vi "ClientRedo.vi"() -> ()   [LabVIEW 2021]
uses:
  20d74f8f-2e8a-4c06-b98a-87e5722cdd8e.vi
  62bce69e-c64b-4137-aa5a-28c05fbbfa3f.vi
  291e4df5-79fb-4e3f-9a4e-f279d7d5f535.vi
  9bb5296f-f4a3-453d-b6f9-cf16bd393dd9.vi
  233518c0-d511-4a3a-97e5-802c987fc087.vi
  913f2bc2-969c-46f7-9a09-9ea84eabe3ee.vi
  <vilib>/Utility/file.llb/Write Delimited Spreadsheet (string).vi
panel:
  in  "file path (dialog if empty)":path=path "D:/APU Stuff/Bachelor of Computer Science (Intelligent Systems) [APD2F2202CS(IS)]/Semester 1/System Programming and Computer Control [CT047-3-2-SPCC]/Assignment/SystemRedo/Zone Status Changes.csv"
  in  "stop":bool
  in  "C6":bool
  in  "C5":bool
  in  "C4":bool
  in  "C3":bool
  in  "C2":bool
  in  "C1":bool
  in  "B6":bool
  in  "B5":bool
  in  "B4":bool
  in  "B3":bool
  in  "B2":bool
  in  "B1":bool
  in  "A6":bool
  in  "A5":bool
  in  "A4":bool
  in  "A3":bool
  in  "A2":bool
  in  "A1":bool
  # "1"
  # "2"
  # "3"
  # "4"
  # "5"
  # "6"
  # "Alarm Switches"
  # "Zone"
  # "Bypass Switches"
  # "Tamper Switches"
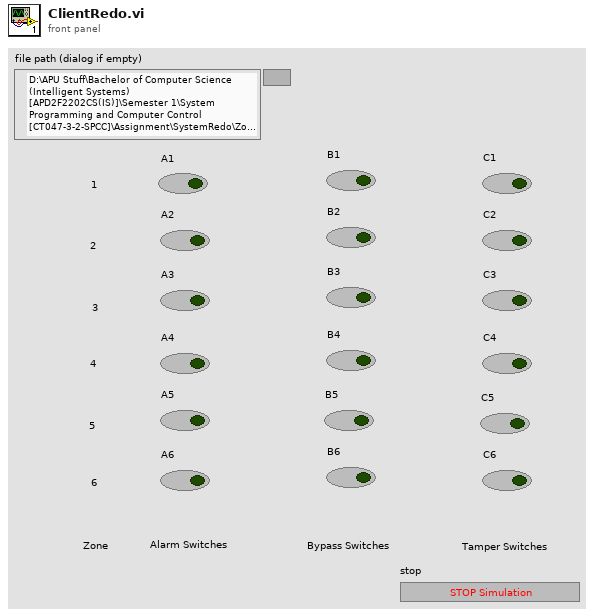
[diagram p1: front panel]
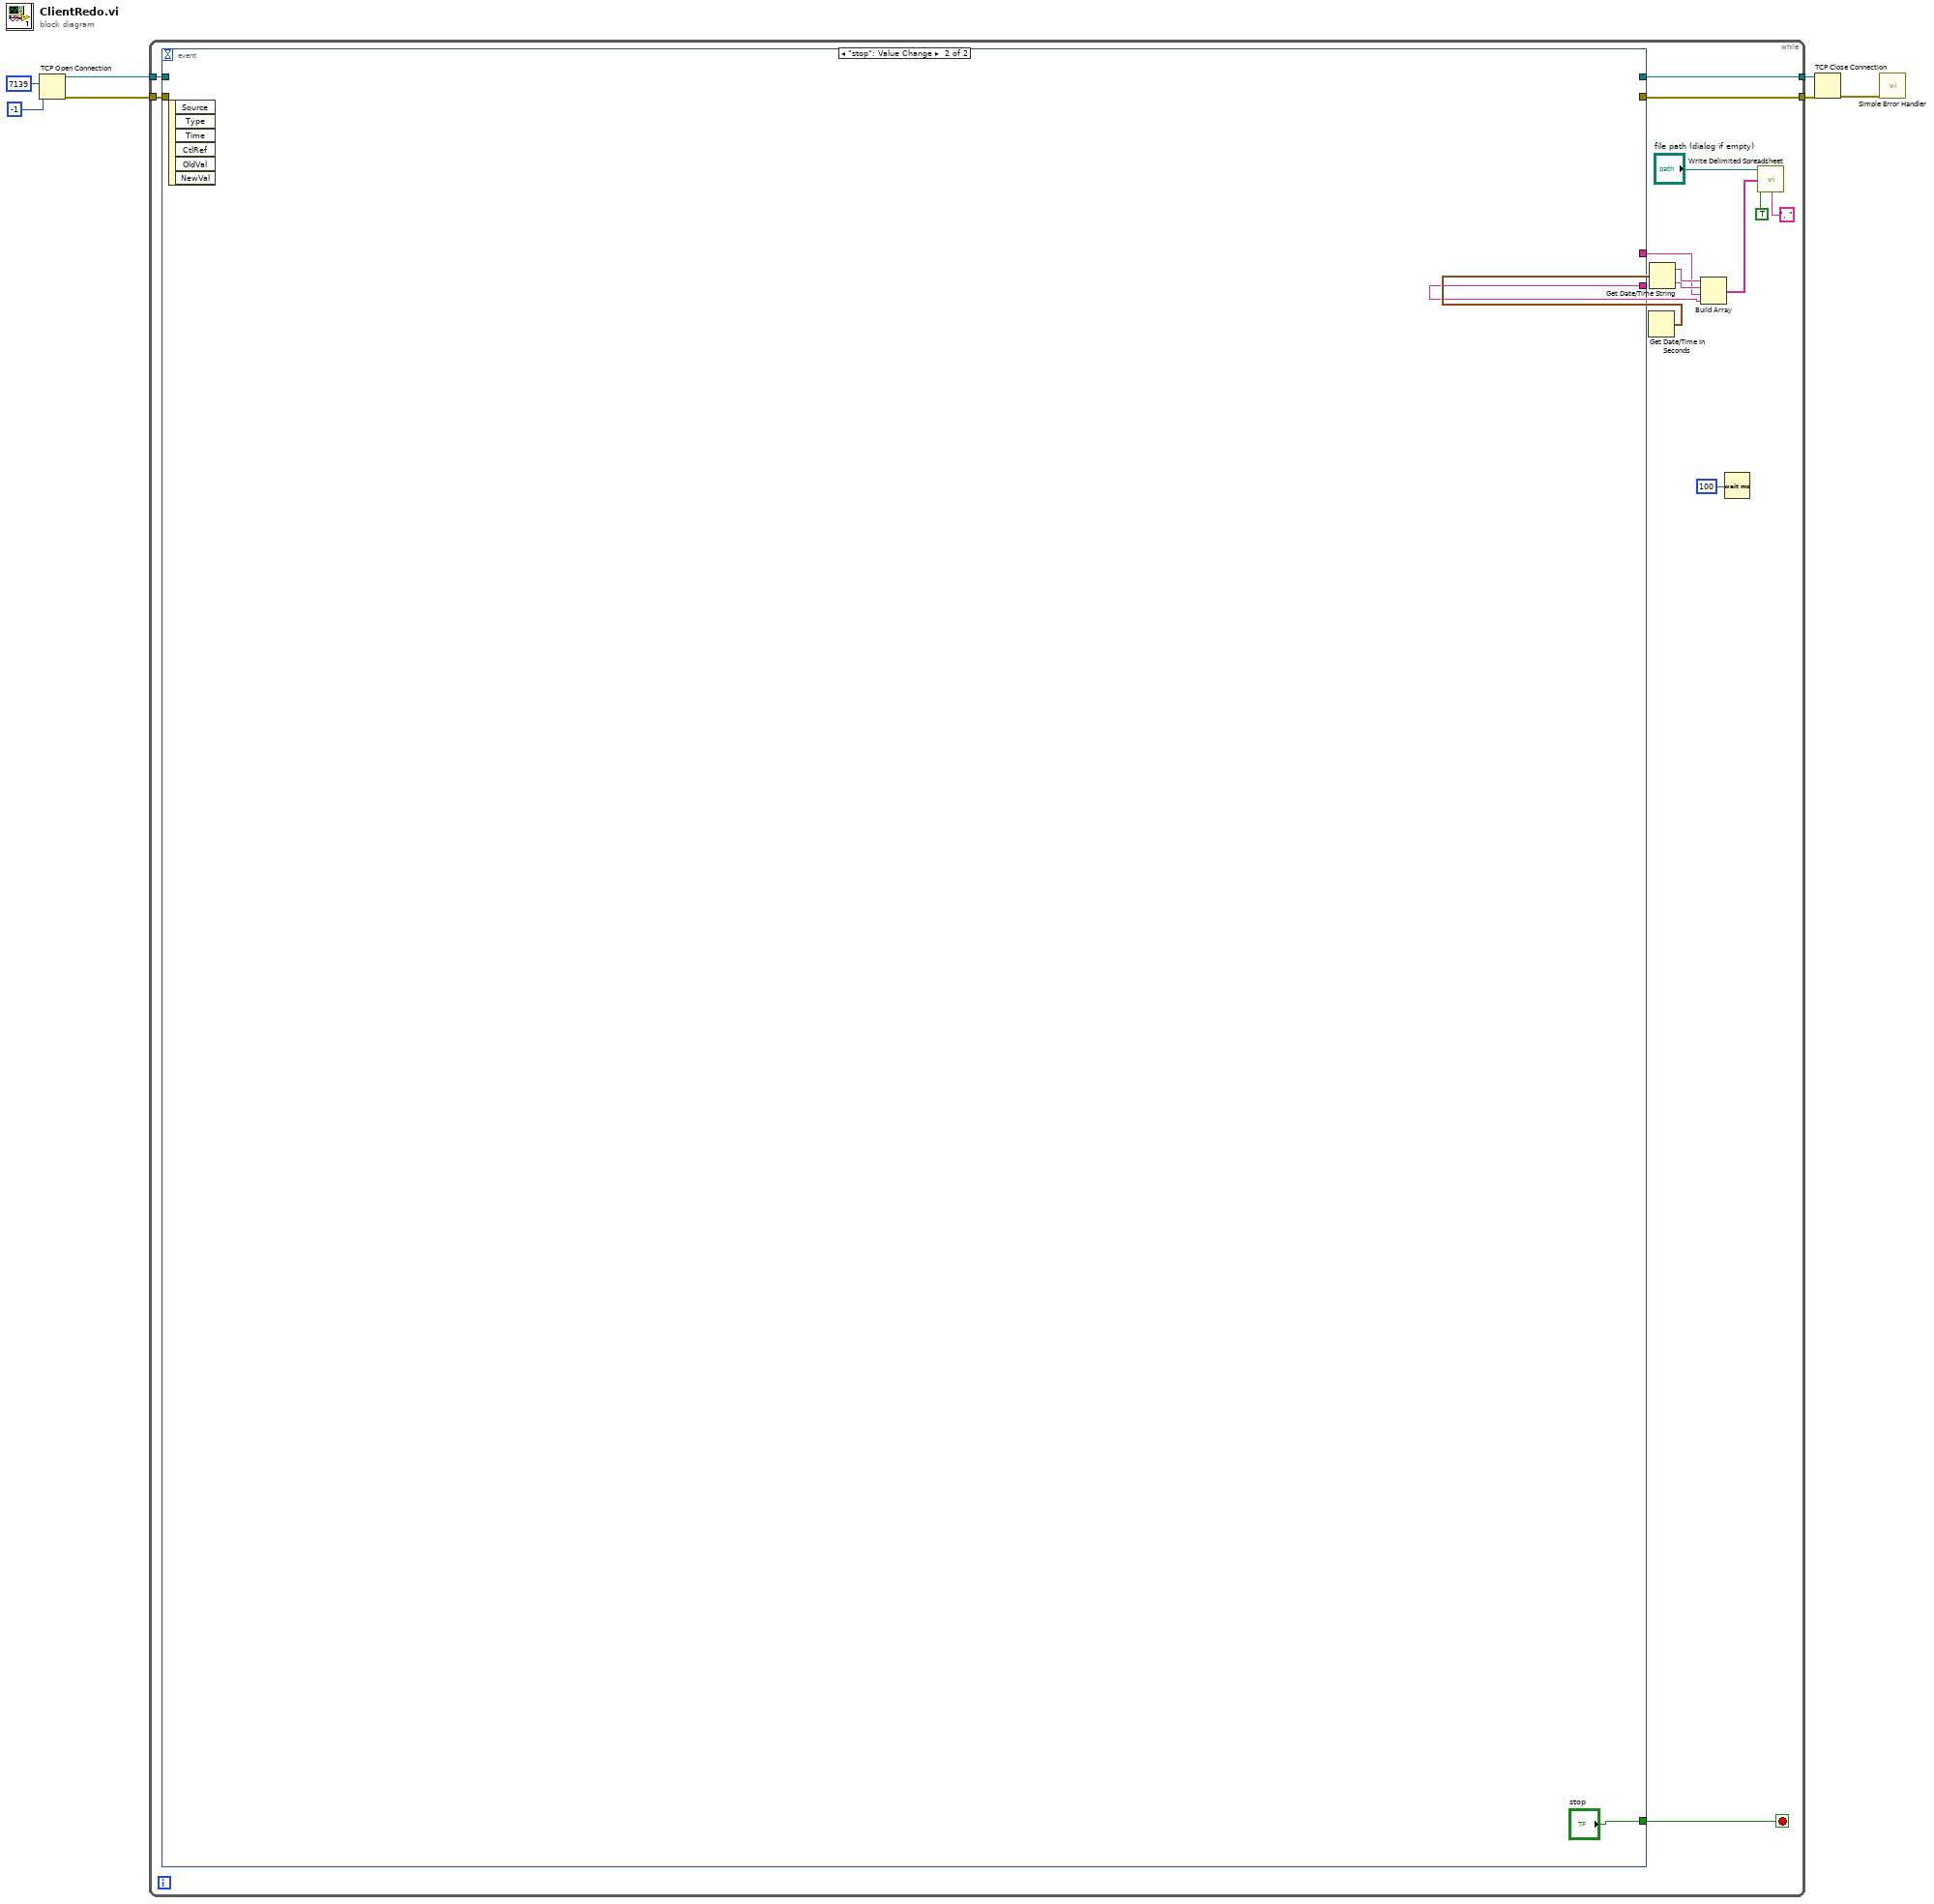
[diagram p0: block diagram]
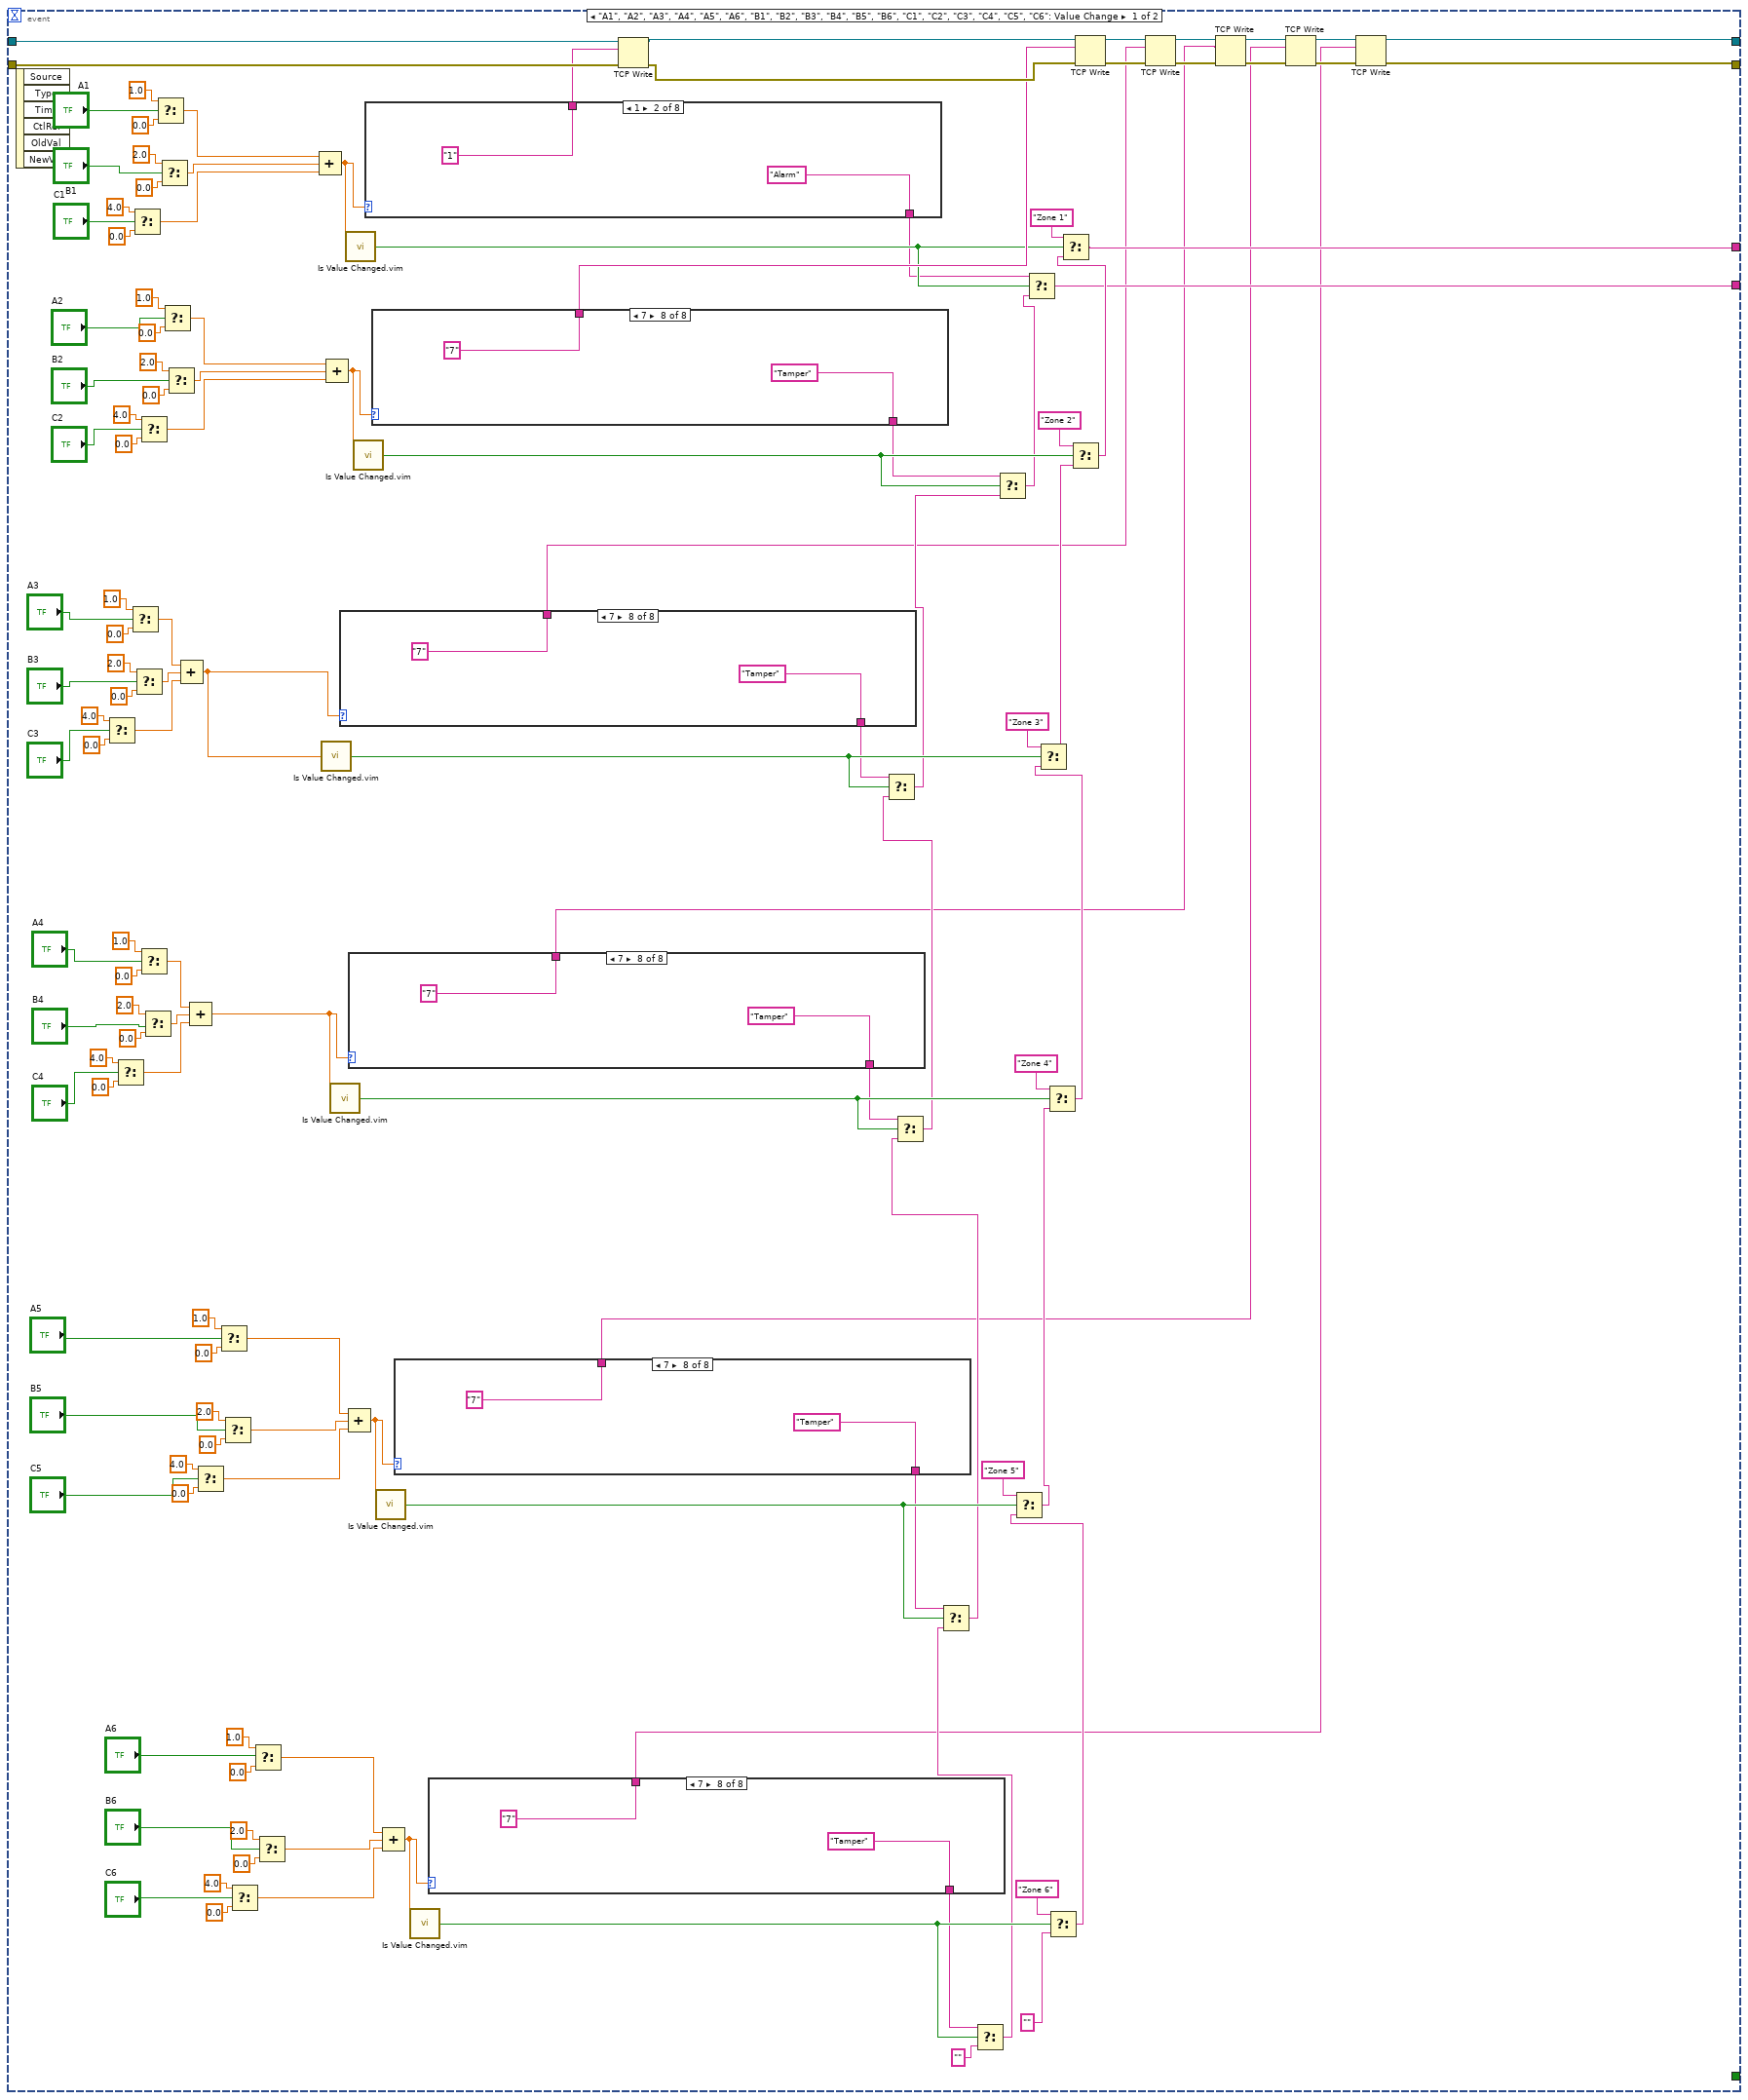
[diagram p2: hidden frame]
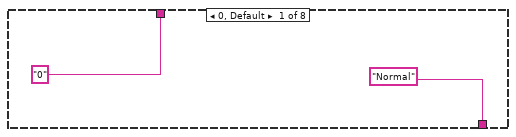
[diagram p3: hidden frame]
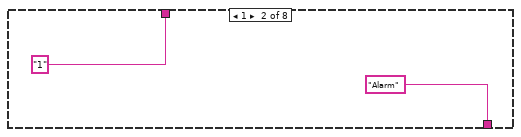
[diagram p4: hidden frame]
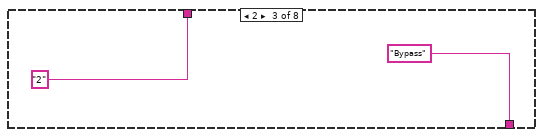
[diagram p5: hidden frame]
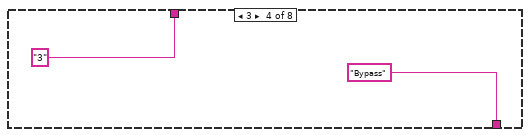
[diagram p6: hidden frame]
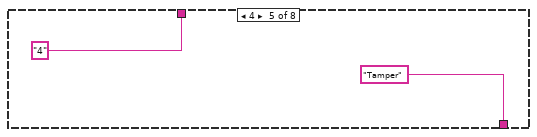
[diagram p7: hidden frame]
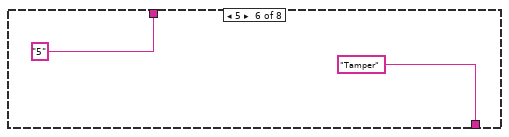
[diagram p8: hidden frame]
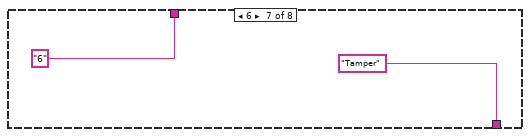
[diagram p9: hidden frame]
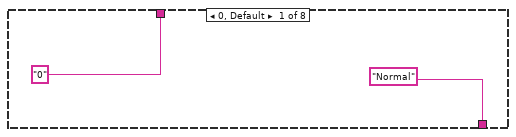
[diagram p10: hidden frame]
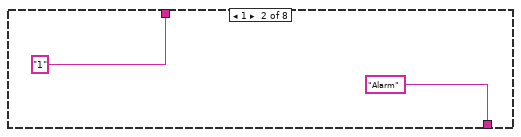
[diagram p11: hidden frame]
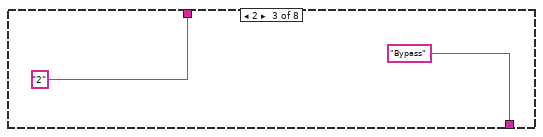
[diagram p12: hidden frame]
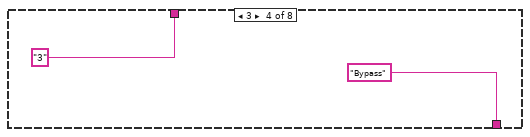
[diagram p13: hidden frame]
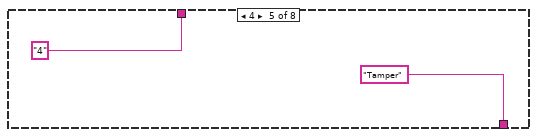
[diagram p14: hidden frame]
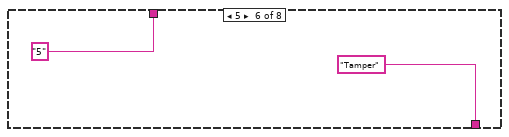
[diagram p15: hidden frame]
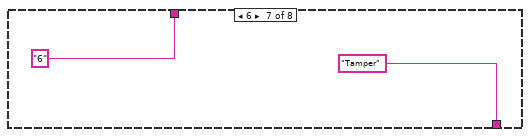
[diagram p16: hidden frame]
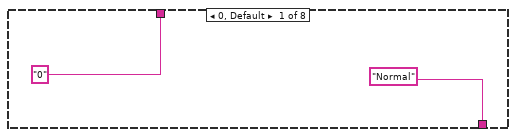
[diagram p17: hidden frame]
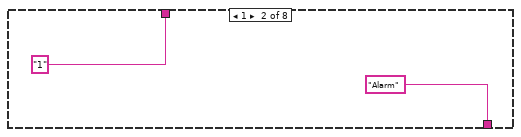
[diagram p18: hidden frame]
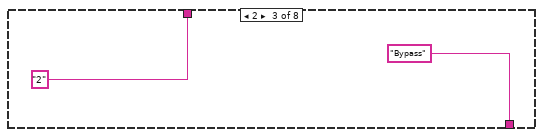
[diagram p19: hidden frame]
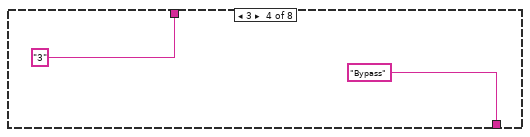
[diagram p20: hidden frame]
diagram:
  n1 = TCP Open Connection(remote port or service name=u16 7139, timeout ms (60000)=-1) -> (connection ID=w7:refnum<k5>, error out=w5:errorcluster)  [unwired: 3 in]
  n2 = while {
    tunnel: w7 -> [w22]
    tunnel: [w19] -> w6
    tunnel: w5 -> [w21]
    tunnel: [w18] -> w4
    stop <- w8 stop-if-true
    n3 = event shown="[1] \"stop\": Value Change" {
      selector: _ -> [_ _]
      dyn-events: _ -> [_ _]
      timeout: _ -> [_ _]
      tunnel: w22 -> [w140 _]
      tunnel: w21 -> [w139 _]
      tunnel: [w86 _] -> w19
      tunnel: [w91 _] -> w18
      tunnel: [w117 _] -> w13
      tunnel: [w111 _] -> w12
      tunnel: [_ "stop"] -> w8
      event "A1", "A2", "A3", "A4", "A5", "A6", "B1", "B2", "B3", "B4", "B5", "B6", "C1", "C2", "C3", "C4", "C5", "C6": Value Change {
        n4 = event-data() -> ()  [unwired: 1 in, 6 out]
        n5 = Select(t=4.0, s="C3", f=0.0) -> (s? t:f=w103:dbl)
        n6 = Select(t=4.0, s="C4", f=0.0) -> (s? t:f=w77:dbl)
        n7 = Select(t=1.0, s="A3", f=0.0) -> (s? t:f=w108:dbl)
        n8 = Select(t=4.0, s="C1", f=0.0) -> (s? t:f=w143:dbl)
        n9 = Select(t=2.0, s="B3", f=0.0) -> (s? t:f=w104:dbl)
        n10 = Select(t=4.0, s="C2", f=0.0) -> (s? t:f=w130:dbl)
        n11 = Select(t=1.0, s="A4", f=0.0) -> (s? t:f=w82:dbl)
        n12 = Select(t=2.0, s="B4", f=0.0) -> (s? t:f=w78:dbl)
        n13 = Select(t=1.0, s="A1", f=0.0) -> (s? t:f=w149:dbl)
        n14 = Select(t=2.0, s="B1", f=0.0) -> (s? t:f=w144:dbl)
        n15 = Select(t=1.0, s="A2", f=0.0) -> (s? t:f=w135:dbl)
        n16 = Select(t=2.0, s="B2", f=0.0) -> (s? t:f=w131:dbl)
        n17 = Compound Arithmetic op=ADD(w108, w104, w103) -> (w101:dbl)
        n18 = Compound Arithmetic op=ADD(w82, w78, w77) -> (w75:dbl)
        n19 = Select(t=4.0, s="C5", f=0.0) -> (s? t:f=w37:dbl)
        n20 = Select(t=1.0, s="A5", f=0.0) -> (s? t:f=w42:dbl)
        n21 = Select(t=2.0, s="B5", f=0.0) -> (s? t:f=w38:dbl)
        n22 = Select(t=4.0, s="C6", f=0.0) -> (s? t:f=w64:dbl)
        n23 = Select(t=1.0, s="A6", f=0.0) -> (s? t:f=w69:dbl)
        n24 = Select(t=2.0, s="B6", f=0.0) -> (s? t:f=w65:dbl)
        n25 = Compound Arithmetic op=ADD(w149, w144, w143) -> (w122:dbl)
        n26 = call "Is Value Changed.vim"("value"=w101) -> ("changed or first call?"=w99:bool)
        n27 = Compound Arithmetic op=ADD(w135, w131, w130) -> (w120:dbl)
        n28 = call "Is Value Changed.vim"("value"=w75) -> ("changed or first call?"=w73:bool)
        n29 = case shown="7" w101 {
          tunnel: ["0" "1" "2" "3" "4" "5" "6" "7"] -> w85
          tunnel: ["Normal" "Alarm" "Bypass" "Bypass" "Tamper" "Tamper" "Tamper" "Tamper"] -> w98
          frame 0, Default {
          }
          frame 1 {
          }
          frame 2 {
          }
          frame 3 {
          }
          frame 4 {
          }
          frame 5 {
          }
          frame 6 {
          }
          frame 7 {
          }
        }
        n30 = call "Is Value Changed.vim"("value"=w122) -> ("changed or first call?"=w116:bool)
        n31 = case shown="7" w75 {
          tunnel: ["0" "1" "2" "3" "4" "5" "6" "7"] -> w48
          tunnel: ["Normal" "Alarm" "Bypass" "Bypass" "Tamper" "Tamper" "Tamper" "Tamper"] -> w72
          frame 0, Default {
          }
          frame 1 {
          }
          frame 2 {
          }
          frame 3 {
          }
          frame 4 {
          }
          frame 5 {
          }
          frame 6 {
          }
          frame 7 {
          }
        }
        n32 = Compound Arithmetic op=ADD(w42, w38, w37) -> (w35:dbl)
        n33 = call "Is Value Changed.vim"("value"=w120) -> ("changed or first call?"=w114:bool)
        n34 = case shown="1" w122 {
          tunnel: ["0" "1" "2" "3" "4" "5" "6" "7"] -> w138
          tunnel: ["Normal" "Alarm" "Bypass" "Bypass" "Tamper" "Tamper" "Tamper" "Tamper"] -> w115
          frame 0, Default {
          }
          frame 1 {
          }
          frame 2 {
          }
          frame 3 {
          }
          frame 4 {
          }
          frame 5 {
          }
          frame 6 {
          }
          frame 7 {
          }
        }
        n35 = case shown="7" w120 {
          tunnel: ["0" "1" "2" "3" "4" "5" "6" "7"] -> w123
          tunnel: ["Normal" "Alarm" "Bypass" "Bypass" "Tamper" "Tamper" "Tamper" "Tamper"] -> w113
          frame 0, Default {
          }
          frame 1 {
          }
          frame 2 {
          }
          frame 3 {
          }
          frame 4 {
          }
          frame 5 {
          }
          frame 6 {
          }
          frame 7 {
          }
        }
        n36 = call "Is Value Changed.vim"("value"=w35) -> ("changed or first call?"=w33:bool)
        n37 = Compound Arithmetic op=ADD(w69, w65, w64) -> (w62:dbl)
        n38 = case shown="7" w35 {
          tunnel: ["0" "1" "2" "3" "4" "5" "6" "7"] -> w24
          tunnel: ["Normal" "Alarm" "Bypass" "Bypass" "Tamper" "Tamper" "Tamper" "Tamper"] -> w32
          frame 0, Default {
          }
          frame 1 {
          }
          frame 2 {
          }
          frame 3 {
          }
          frame 4 {
          }
          frame 5 {
          }
          frame 6 {
          }
          frame 7 {
          }
        }
        n39 = call "Is Value Changed.vim"("value"=w62) -> ("changed or first call?"=w59:bool)
        n40 = case shown="7" w62 {
          tunnel: ["0" "1" "2" "3" "4" "5" "6" "7"] -> w23
          tunnel: ["Normal" "Alarm" "Bypass" "Bypass" "Tamper" "Tamper" "Tamper" "Tamper"] -> w58
          frame 0, Default {
          }
          frame 1 {
          }
          frame 2 {
          }
          frame 3 {
          }
          frame 4 {
          }
          frame 5 {
          }
          frame 6 {
          }
          frame 7 {
          }
        }
        n41 = TCP Write(connection ID=w140, data in=w138, error in (no error)=w139) -> (connection ID out=w125:refnum<k5>, error out=w124:errorcluster)  [unwired: 1 in, 1 out]
        n42 = Select(t=w58, s=w59, f="") -> (s? t:f=w25:string)
        n43 = Select(t=w32, s=w33, f=w25) -> (s? t:f=w27:string)
        n44 = Select(t=w72, s=w73, f=w27) -> (s? t:f=w49:string)
        n45 = Select(t=w98, s=w99, f=w49) -> (s? t:f=w96:string)
        n46 = Select(t=w113, s=w114, f=w96) -> (s? t:f=w112:string)
        n47 = Select(t=w115, s=w116, f=w112) -> (s? t:f=w111:string)
        n48 = Select(t="Zone 6", s=w59, f="") -> (s? t:f=w26:string)
        n49 = Select(t="Zone 5", s=w33, f=w26) -> (s? t:f=w28:string)
        n50 = Select(t="Zone 4", s=w73, f=w28) -> (s? t:f=w50:string)
        n51 = Select(t="Zone 3", s=w99, f=w50) -> (s? t:f=w97:string)
        n52 = Select(t="Zone 2", s=w114, f=w97) -> (s? t:f=w118:string)
        n53 = Select(t="Zone 1", s=w116, f=w118) -> (s? t:f=w117:string)
        n54 = TCP Write(connection ID=w125, data in=w123, error in (no error)=w124) -> (connection ID out=w90:refnum<k5>, error out=w95:errorcluster)  [unwired: 1 in, 1 out]
        n55 = TCP Write(connection ID=w90, data in=w85, error in (no error)=w95) -> (connection ID out=w89:refnum<k5>, error out=w94:errorcluster)  [unwired: 1 in, 1 out]
        n56 = TCP Write(connection ID=w89, data in=w48, error in (no error)=w94) -> (connection ID out=w88:refnum<k5>, error out=w93:errorcluster)  [unwired: 1 in, 1 out]
        n57 = TCP Write(connection ID=w88, data in=w24, error in (no error)=w93) -> (connection ID out=w87:refnum<k5>, error out=w92:errorcluster)  [unwired: 1 in, 1 out]
        n58 = TCP Write(connection ID=w87, data in=w23, error in (no error)=w92) -> (connection ID out=w86:refnum<k5>, error out=w91:errorcluster)  [unwired: 1 in, 1 out]
      }
      event "stop": Value Change {
        n59 = event-data() -> ()  [unwired: 1 in, 6 out]
      }
    }
    n60 = Get Date/Time In Seconds() -> (seconds since 1Jan1904=w14:timestamp)
    n61 = Get Date/Time String(seconds (now)=w14) -> (date string=w16:string, time string=w15:string)  [unwired: 2 in]
    n62 = Build Array(w16, w15, w13, w12) -> (w11:string[])
    n63 = Wait (ms)(milliseconds to wait=u32 100) -> ()  [unwired: 1 out]
    n64 = call-poly <vilib>:"Write Delimited Spreadsheet.vi"("file path (dialog if empty)"="file path (dialog if empty)", "1D data"=w11, "append to file? (new file:F)"=TRUE, "delimiter (\\t)"=", " ("delimiter (\\t)")) -> ()  [unwired: 10 in, 2 out]
  }
  n65 = TCP Close Connection(connection ID=w6, error in (no error)=w4) -> (error out=w1:errorcluster)  [unwired: 1 in, 1 out]
  n66 = call <vilib>:"Simple Error Handler.vi"("error in (no error)"=w1) -> ()  [unwired: 4 in, 5 out]
